vi "wavefunction.vi"() -> ()   [LabVIEW 2019]
uses:
  <vilib>/measure/NI_MABase.lvlib
panel:
  in  "signal type":T1(ring)
  in  "stop":bool
  out "Waveform Graph":waveform(dbl)(graph)
  in  "phase":dbl
  in  "f":dbl(knob) scale=0.0..10.0
  in  "A":dbl(knob) scale=0.0..10.0
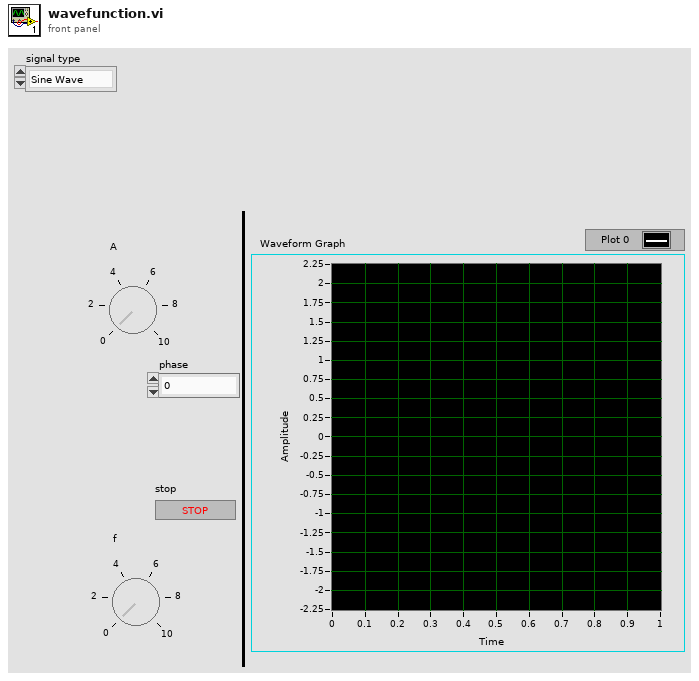
[diagram p1: front panel]
types:
  T1 = enum16{"Sine Wave", "Triangle Wave", "Square Wave", "Sawtooth Wave"}
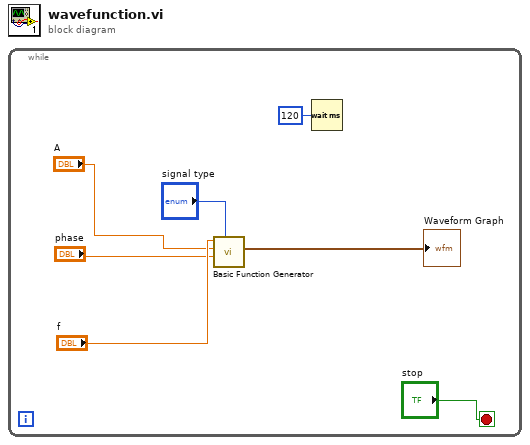
[diagram p0: block diagram]
diagram:
  n1 = while {
    stop <- "stop" stop-if-true
    n2 = call <vilib>:"Basic Function Generator.vi"("signal type"="signal type", "phase"="phase", "amplitude"="A", "frequency"="f") -> ("signal out"=→"Waveform Graph":waveform(dbl))  [unwired: 5 in, 2 out]
    n3 = Wait (ms)(milliseconds to wait=u32 120) -> ()  [unwired: 1 out]
  }
